vi "GetNI_SaveToFile_25_AVG.vi"(0 "Digitizer Settings":T4={"Digitizer delay (us) "=0.0, "rf points per line"=2048, "lines per plane"=128, "Samp Rate (Hz)"=100000000.0, "Additional dig delay (us)"=0.0, "Voltage Scale"=0.4, "Pre-Looks"=0, "Offset delay (us)"=0.0, "bits A/D"=8, "Avg Num"=1, "DigTimeOut"=5.0, "Rel Dig Delay"=0.0, "Dig Ch"=0, "LeCroyCluster"={"LeCroy Channels"=[TRUE, FALSE, FALSE, FALSE], "LC read pt offset"=0.0, "Sweep Avg"=FALSE}, "Main Digitizer"=enum."NI Digitizer", "Dig Config"=enum."Single channel", "Digitizer ID Cluster"={"Acqiris/Alazar/SP ID"=[], "NI Instr Handles"=[], "LeCroy VISA"="", "GaGe Handle"={"Handle"=0, "Sample size"=0, "Resolution"=0, "Offset"=0, "Channels"=0, "Boards"=0}, "ATS Ref"="ATS9350", "Acqiris Address"=["PCI::INSTR0"], "ADQRef"=refnum, "adq_cu_ptr"=refnum}, "Trigger Settings"={"Trig Source"=1, "Trig Coupling"=0, "Trig Slope"=0, "Level (mV)"=1500.0}, "Bulk Acq"=FALSE, "Bulk Start Indexes"=[], "Data Ref RF"=refnum, "NI ID/Channel"=[], "Total Dig CH"=1, "Xtra Ann Trig delay (us)"=10.0, "Fix Z Delay?"=FALSE, "One Way Transmission?"=FALSE, "Data Ref Log"=refnum} {"Trigger Settings"."Trig Slope" items=["Positive", "Negative"]; "Trigger Settings"."Level (mV)" format="%.2f"; "Trigger Settings"."Trig Coupling" items=["DC 1 MOhm", "AC 1 MOhm", "DC 50 Ohm", "AC 50 Ohm"]; "Trigger Settings"."Trig Source" items=["Chan 1", "External"]; "Rel Dig Delay" format="%.2f"; "DigTimeOut" format="%.2f"; "Avg Num" min=1; "Offset delay (us)" format="%.2f"; "Additional dig delay (us)" format="%.2f"; "Digitizer delay (us)" format="%.2f"}, 3 "Ann Array Params":T1={"Synth Foc?"=FALSE, "Focal Zones"=41, "Switch T/R"=0, "Trans Geometry (mm)"={"Transducer"=0, "Geo Focus"=12.0, "a (radius)"=3.0, "# of rings"=5, "kerf space "=0.1, "Center Freq"=12.0}, "Sub Ap Excite?"=FALSE, "Full Array Scan?"=FALSE, "Xmt/Rcv"={"XMIT"=[TRUE, TRUE, TRUE, TRUE, TRUE], "RCV"=[TRUE, TRUE, TRUE, TRUE, TRUE]}, "PulseSpacing (us)"=0.0, "Xmit Ring"=0, "XMIT CHS"=0, "RCV CHS"=0, "GPU?"=FALSE, "Save TIFF?"=FALSE, "downfactor"=1, "RCV 1CH"=0} {"RCV 1CH" items=["All", "1", "2", "3", "4", "5"]; "Trans Geometry (mm)"."Transducer" items=["6D 12R 40 MHz"=0, "10D 31R 20 MHz"=1, "10D 23R 20 MHz"=2, "6D 23R 40 MHz"=3, "4.5D 10.7R 40 MHz"=4, "9D 23.5R 20 MHz"=5, "9D 25.8R 20MHz"=6, "Enter"=99]; "Switch T/R" min=1 max=5 step=1}, 7 "errorin":errorcluster, 8 "File Array":string[](array[string]), 10 "lines per plane":i32) -> (17 "Raw VGain (scale)":dbl, 18 "Gain Array":T8(array[cluster]), 20 "data out":i8[][][](array[numeric]), 21 "VGain (dB)":dbl, 27 "error out":errorcluster)   [LabVIEW 2022 SP3]
uses:
  -DigitizerRoutines/DigitizerSettings.ctl
  -DigitizerRoutines/Digitizer.ctl
  -DigitizerRoutines/DigConfig.ctl
  -DigitizerRoutines/DigitizerID.ctl
  C:/Windows/System32/ADQAPI_dotNet_helper.dll
  Annular Array/-AnnularRoutines/AnnularArray.ctl
  Annular Array/-AnnularRoutines/TransGeometry.ctl
  Annular Array/-AnnularRoutines/ArrayGeometry.ctl
  <instrlib>/niScope/Acquire/Fetch/niScope Multi Fetch Binary 8.vi
panel:
  out "read time":u32
  out "save time":u32
  out "Numeric":i32
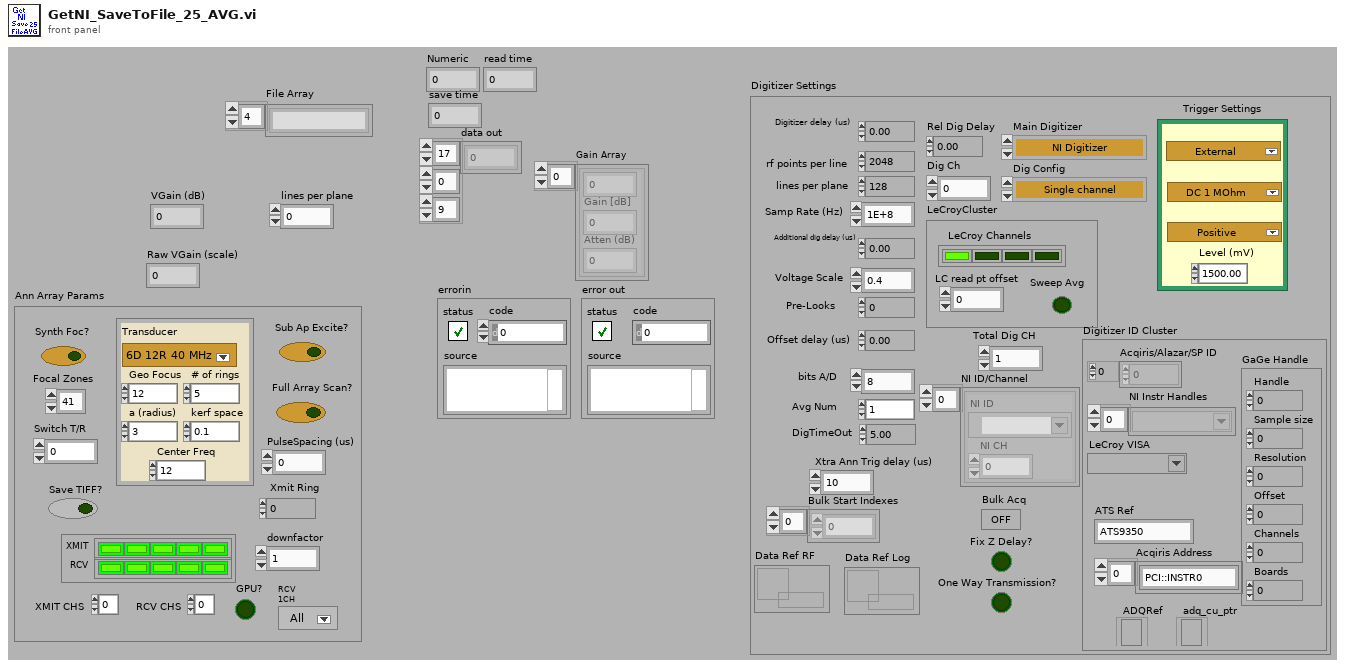
[diagram p1: front panel]
types:
  T1 = typedef "AnnularArray.ctl" = cluster{"Synth Foc?":bool, "Focal Zones":i16, "Switch T/R":i16, "Trans Geometry (mm)":T2, "Sub Ap Excite?":bool, "Full Array Scan?":bool, "Xmt/Rcv":cluster{"XMIT":bool[], "RCV":bool[]}, "PulseSpacing (us)":sgl, "Xmit Ring":i32, "XMIT CHS":u8, "RCV CHS":u8, "GPU?":bool, "Save TIFF?":bool, "downfactor":i32, "RCV 1CH":u16}
  T2 = typedef "TransGeometry.ctl" = cluster{"Transducer":T3, "Geo Focus":dbl, "a (radius)":dbl, "# of rings":i32, "kerf space ":dbl, "Center Freq":dbl}
  T3 = typedef "ArrayGeometry.ctl" = u16
  T4 = typedef "DigitizerSettings.ctl" = cluster{"Digitizer delay (us) ":dbl, "rf points per line":i32, "lines per plane":i32, "Samp Rate (Hz)":dbl, "Additional dig delay (us)":dbl, "Voltage Scale":dbl, "Pre-Looks":i32, "Offset delay (us)":dbl, "bits A/D":i8, "Avg Num":i32, "DigTimeOut":sgl, "Rel Dig Delay":sgl, "Dig Ch":i32, "LeCroyCluster":cluster{"LeCroy Channels":bool[], "LC read pt offset":dbl, "Sweep Avg":bool}, "Main Digitizer":T5, "Dig Config":T6, "Digitizer ID Cluster":T7, "Trigger Settings":cluster{"Trig Source":u16, "Trig Coupling":u16, "Trig Slope":u16, "Level (mV)":dbl}, "Bulk Acq":bool, "Bulk Start Indexes":i32[], "Data Ref RF":refnum<data-value>, "NI ID/Channel":cluster{"NI ID":refnum<k15>, "NI CH":i32}[], "Total Dig CH":i32, "Xtra Ann Trig delay (us)":dbl, "Fix Z Delay?":bool, "One Way Transmission?":bool, "Data Ref Log":refnum<data-value>}
  T5 = typedef "Digitizer.ctl" = enum16{"Acqiris Digitizer", "NI Digitizer", "LeCroy", "GaGe", "AlazarTech", "No Digitizer", "Teledyne"}
  T6 = typedef "DigConfig.ctl" = enum16{"Single channel", "2 Chans w/ 2 Acqiris", "2 Chans w/ 1 Acqiris", "5-CH Pulser New", "5-CH pulser w/ ann array", "5-pass style ann array", "Empty"}
  T7 = typedef "DigitizerID.ctl" = cluster{"Acqiris/Alazar/SP ID":u32[], "NI Instr Handles":refnum<k15>[], "LeCroy VISA":refnum<visa-resource-name>, "GaGe Handle":cluster{"Handle":u32, "Sample size":u32, "Resolution":i32, "Offset":i32, "Channels":u32, "Boards":u32}, "ATS Ref":string, "Acqiris Address":string[], "ADQRef":refnum<k24>, "adq_cu_ptr":refnum<k24>}
  T8 = cluster{sgl, "Gain [dB]  ":sgl, "Atten (dB)":sgl}[]
  T9 = cluster{"gain":dbl, "wfm":i8[][], "max queue size (-1, unlimited)":i32}
  T10 = cluster{"actualSamples":i32, "absoluteInitialX":dbl, "relativeInitialX":dbl, "xIncrement":dbl, "offset":dbl, "gain":dbl, "reserved1":dbl, "reserved2":dbl}[]
  T11 = cluster{"actualSamples":i32, "absoluteInitialX":dbl, "relativeInitialX":dbl, "xIncrement":dbl, "offset":dbl, "gain":dbl, "reserved1":dbl, "reserved2":dbl}
  T12 = cluster{sgl, "Gain [dB]  ":sgl, "Atten (dB)":sgl}
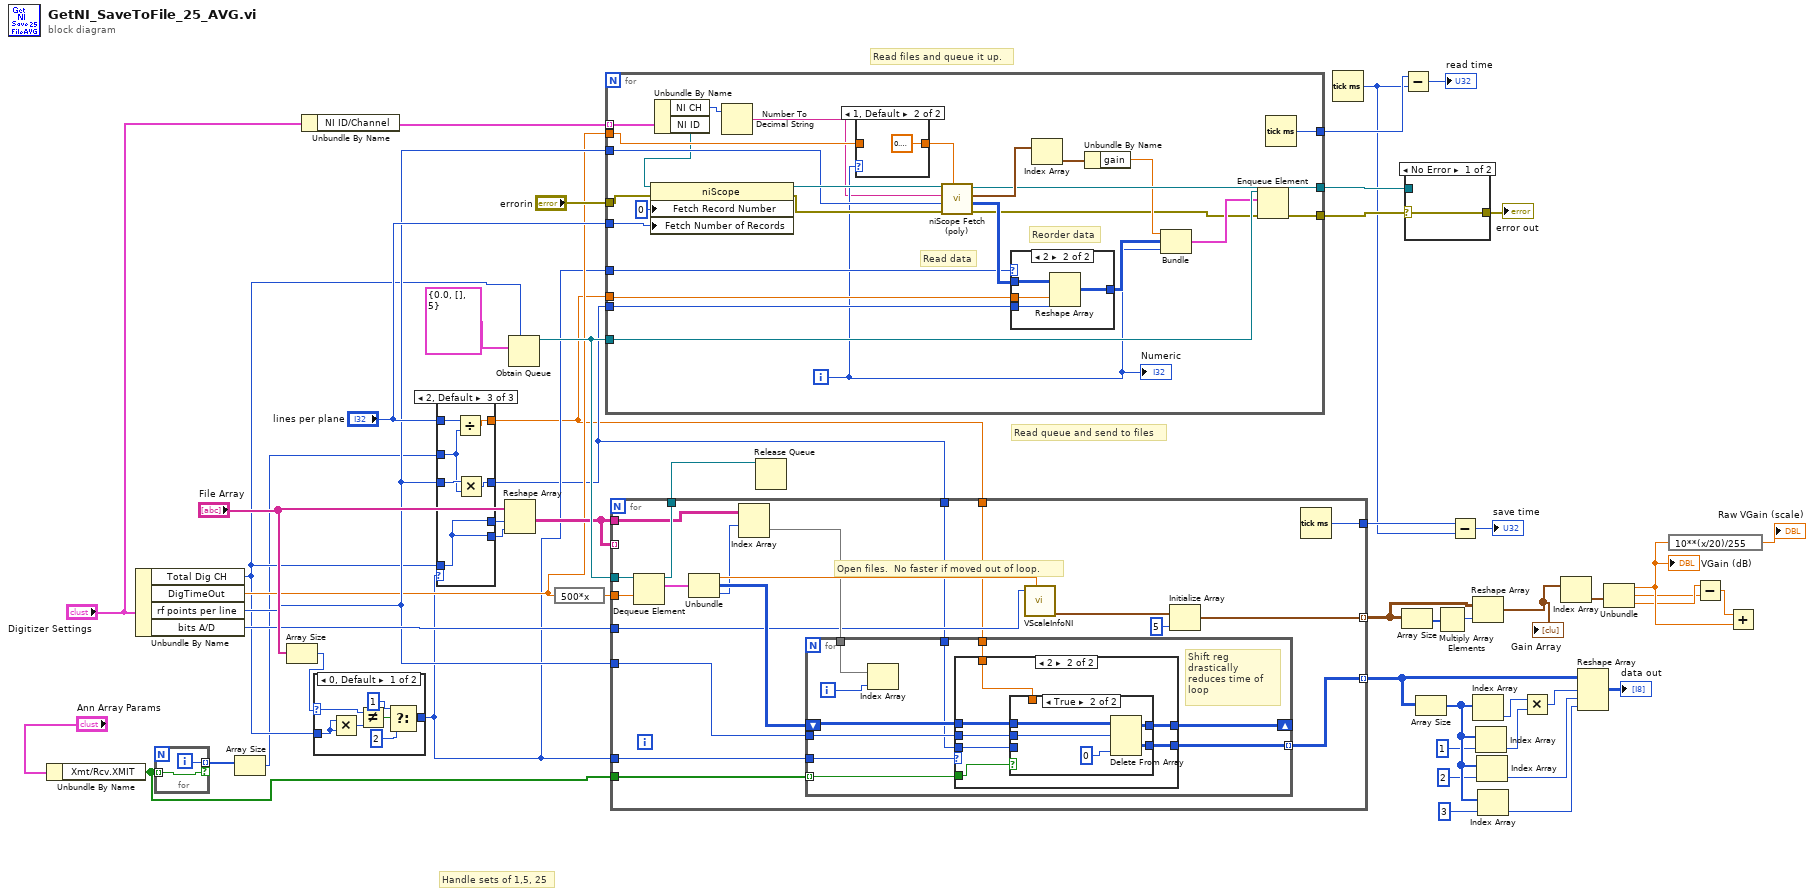
[diagram p0: block diagram]
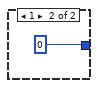
[diagram p2: hidden frame]
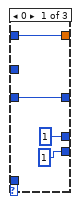
[diagram p3: hidden frame]
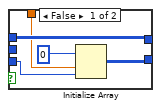
[diagram p6: hidden frame]
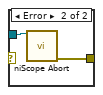
[diagram p7: hidden frame]
diagram:
  # "Handle sets of 1,5, 25"
  # "Read files and queue it up."
  # "Read queue and send to files"
  n1 = Unbundle By Name("Ann Array Params") -> ("Xmt/Rcv.XMIT"=w3:bool[])
  n2 = Unbundle By Name("Digitizer Settings") -> ("Total Dig CH"=w8:i32, "DigTimeOut"=w12:sgl, "rf points per line"=w13:i32, "bits A/D"=w14:i8)
  n3 = for {
    tunnel: w3 -> [w54] mode=indexing
    tunnel: [w55] -> w5 mode=indexing if=w54
    i -> [w55]
  }
  n4 = Array Size(array=w5) -> (size(s)=w4:i32)
  n5 = Array Size(array="File Array") -> (size(s)=w9:i32)
  n6 = Unbundle By Name("Digitizer Settings") -> ("NI ID/Channel"=w10:cluster{"NI ID":refnum<k15>, "NI CH":i32}[])
  n7 = case shown="0, Default" w9 {
    selector: w9 -> [w62 _]
    tunnel: [w61 0] -> w7
    tunnel: w8 -> [w56 _]
    frame 0, Default {
      n8 = Multiply(x=w56, y=w56) -> (x*y=w59:i32)
      n9 = Not Equal?(x=w62, y=w59) -> (x != y?=w60:bool)
      n10 = Select(t=1, s=w60, f=2) -> (s? t:f=w61:i32)
    }
    frame 1 {
    }
  }
  n11 = case shown="2, Default" w7 {
    tunnel: [1 w68 w73] -> w34
    tunnel: [w66 w70 w76] -> w2
    tunnel: w13 -> [w66 w70 w75]
    tunnel: [w65 w69 w72] -> w1
    tunnel: "lines per plane" -> [w65 w69 w74]
    tunnel: [1 w68 w73] -> w32
    tunnel: w8 -> [_ w68 w73]
    tunnel: w4 -> [_ _ w71]
    frame 0 {
    }
    frame 1 {
    }
    frame 2, Default {
      n12 = Divide(x=w74, y=w71) -> (x/y=w72:dbl)
      n13 = Multiply(x=w75, y=w71) -> (x*y=w76:i32)
    }
  }
  n14 = Reshape Array("File Array", w34, w32) -> (w30:string[][])
  n15 = Obtain Queue(max queue size (-1, unlimited)=w8, element data type=T9 {"gain"=0.0, "wfm"=[], "max queue size (-1, unlimited)"=5}) -> (queue out=w43:refnum<queue>)  [unwired: 3 in, 2 out]
  n16 = expression code="500*x"(w12) -> (w31:sgl)
  n17 = for {
    tunnel: w12 -> [w83]
    tunnel: w13 -> [w95]
    tunnel: "errorin" -> [w103]
    tunnel: "lines per plane" -> [w98]
    tunnel: [w97] -> w51
    tunnel: w43 -> [w94]
    tunnel: [w84] -> w42
    tunnel: [w91] -> w41
    tunnel: w1 -> [w89]
    tunnel: w2 -> [w88]
    tunnel: w7 -> [w87]
    tunnel: w10 -> [w80] mode=indexing
    i -> [w81]
    # "Reorder data"
    # "Read data"
    n18 = Unbundle By Name(w80) -> ("NI CH"=w78:i32, "NI ID"=w79:refnum<k15>)
    n19 = property class="niScope"(reference=w79, error in=w103, "Fetch Record Number"=0, "Fetch Number of Records"=w98) -> (reference out=w96:refnum<k15>, error out=w102:errorcluster)
    n20 = Number To Decimal String(number=w78) -> (decimal integer string=w77:string)  [unwired: 1 out]
    n21 = case shown="1, Default" w81 {
      tunnel: w83 -> [w104 _]
      tunnel: [w104 sgl 0.1 ("DigTimeOut")] -> w82
      frame 0 {
      }
      frame 1, Default {
      }
    }
    n22 = call-poly <instrlib>:"niScope Fetch (poly).vi"("timeout"=w82, "error in"=w102, "numSamples"=w95, "channels"=w77, "instrument handle"=w96) -> ("error out"=w85:errorcluster, "wfm"=w90:i8[][], "wfm info"=w101:T10, "instrument handle out"=w97:refnum<k15>)  [unwired: 3 out]
    n23 = case shown="2" w87 {
      tunnel: w88 -> [_ w110]
      tunnel: w90 -> [w106 w109]
      tunnel: [w106 w108] -> w86
      tunnel: w89 -> [_ w107]
      frame 0, Default {
      }
      frame 2 {
        n24 = Reshape Array(w109, w107, w110) -> (w108:i8[][])
      }
    }
    n25 = Index Array(array=w101) -> (element=w100:T11)  [unwired: 1 in]
    n26 = Unbundle By Name(w100) -> ("gain"=w93:dbl)
    n27 = Bundle("gain"=w93, "wfm"=w86, w81) -> (w92:cluster{"gain":dbl, "wfm":i8[][], i32})  [unwired: 1 in]
    n28 = Enqueue Element(queue=w94, element=w92, error in (no error)=w85) -> (error out=w84:errorcluster)  [unwired: 1 in, 2 out]
    n29 = Tick Count (ms)() -> (millisecond timer value=w91:u32)
    "Numeric" <- w81
  }
  n30 = for {
    tunnel: w13 -> [w130]
    tunnel: w30 -> [_] mode=indexing
    tunnel: w43 -> [w129]
    tunnel: [w126] -> w36
    tunnel: [w125] -> w40
    tunnel: w7 -> [w124]
    tunnel: w31 -> [w122]
    tunnel: w30 -> [w121]
    tunnel: [w118] -> w29 mode=indexing
    tunnel: [w115] -> w16 mode=indexing
    tunnel: w14 -> [w114]
    tunnel: w3 -> [w113]
    tunnel: w2 -> [w112]
    tunnel: w1 -> [w111]
    # "Open files.  No faster if moved out of loop."
    n31 = Dequeue Element(queue=w129, timeout in ms (-1)=w122) -> (queue out=w126:refnum<queue>, element=w128:T9)  [unwired: 1 in, 2 out]
    n32 = Unbundle(w128) -> ("gain"=w127:dbl, "wfm"=w123:i8[][], "max queue size (-1, unlimited)"=w120:i32)
    n33 = Index Array(array=w121, index (row)=w120) -> (element=w119:string[])  [unwired: 1 in]
    n34 = for {
      tunnel: w119 -> [w132]
      tunnel: w130 -> [w140]
      tunnel: w124 -> [w138]
      shift-right: [w137] -> _
      shift-left: w123 -> [w139]
      tunnel: [w136] -> w118 mode=indexing
      tunnel: w113 -> [w135] mode=indexing
      tunnel: w112 -> [w134]
      tunnel: w111 -> [w133]
      i -> [w131]
      # "Shift reg drastically reduces time of loop"
      n35 = Index Array(array=w132, index=w131) -> ()  [unwired: 1 out]
      n36 = case shown="2" w138 {
        tunnel: [w141 w145] -> w136
        tunnel: w140 -> [_ w146]
        tunnel: w139 -> [w141 w148]
        tunnel: [w141 w147] -> w137
        tunnel: w135 -> [_ w144]
        tunnel: w134 -> [_ w143]
        tunnel: w133 -> [_ w142]
        frame 5, Default {
        }
        frame 2 {
          n37 = case shown="True" w144 {
            tunnel: w148 -> [w153 w158]
            tunnel: [w153 w157] -> w147
            tunnel: w146 -> [_ w156]
            tunnel: [w152 w154] -> w145
            tunnel: w143 -> [w150 _]
            tunnel: w142 -> [w149 _]
            frame False {
              n38 = Initialize Array(i8 0, w149, w150) -> (w152:i8[][])
            }
            frame True {
              n39 = Delete From Array(array=w158, length=w156, index (col)=0 ("index (row)")) -> (deleted portion=w154:i8[][], array with subset deleted=w157:i8[][])  [unwired: 1 in]
            }
          }
        }
      }
    }
    n40 = call "VScaleInfoNI.vi"("A/D bits"=w114, "gain"=w127) -> ("Voltage Scale"=w116:T12)  [unwired: 5 in, 3 out]
    n41 = Initialize Array(w116, i8 5 ("Atten (dB)")) -> (w115:T8)
    n42 = Tick Count (ms)() -> (millisecond timer value=w125:u32)
  }
  n43 = Release Queue(queue=w36) -> ()  [unwired: 2 in, 3 out]
  n44 = Tick Count (ms)() -> (millisecond timer value=w39:u32)
  n45 = Array Size(array=w16) -> (size(s)=w18:i32[])
  n46 = Subtract(x=w41, y=w39) -> (x-y=→"read time":u32)
  n47 = case shown="No Error" w42 {
    selector: w42 -> [w159 _]
    tunnel: w51 -> [_ w161]
    tunnel: [w159 w160] -> w52
    frame No Error {
    }
    frame Error {
      n48 = call <instrlib>:"niScope Abort.vi"("instrument handle"=w161) -> ("error out"=w160:errorcluster)  [unwired: 1 in, 13 out]
    }
  }
  "error out" <- w52
  n49 = Array Size(array=w29) -> (size(s)=w28:i32[])
  n50 = Multiply Array Elements(1:w18) -> (0:w17:i32)
  n51 = Subtract(x=w40, y=w39) -> (x-y=→"save time":u32)
  n52 = Reshape Array(w16, w17) -> (w15:T8)
  "Gain Array" <- w15
  n53 = Index Array(array=w28) -> (element=w24:i32)  [unwired: 1 in]
  n54 = Index Array(array=w28, index=1) -> (element=w25:i32)
  n55 = Index Array(array=w28, index=2) -> (element=w27:i32)
  n56 = Index Array(array=w28, index=3) -> (element=w26:i32)
  n57 = Multiply(x=w24, y=w25) -> (x*y=w23:i32)
  n58 = Index Array(array=w15) -> (element=w50:T12)  [unwired: 1 in]
  n59 = Reshape Array(w29, w23, w27, w26) -> (→"data out":i8[][][])
  n60 = Unbundle(w50) -> (w49:sgl, "Gain [dB]"=w47:sgl, "Atten (dB)"=w48:sgl)
  "VGain (dB)" <- w49
  n61 = expression code="10**(x/20)/255"(w49) -> (→"Raw VGain (scale)":sgl)
  n62 = Subtract(x=w48, y=w47) -> (x-y=w46:sgl)
  n63 = Add(x=w46, y=w49) -> ()  [unwired: 1 out]
